vi "(SubVI) Trigger and Record Sine Wave_PI_YCC.vi"(6 "Record time (s)":dbl=0.4, 7 "Amplitude (nm)":dbl=1000.0, 8 "freq. (Hz)":dbl=32.0, 9 "Axis  (Enum)":enum16{"x", "y", "z"}(ring)) -> (0 "Start Position (um)":dbl format="%0.5f", 1 "Read Positions Array (um)":dbl[](array[numeric]), 2 "Target Positions Array (um)":dbl[](array[numeric]), 3 "Time Array (s)":dbl[](array[numeric]), 4 "DAC rate (Hz)":dbl=20000.0)   [LabVIEW 2014]
panel:
  out "Axis Array":i32[](array[numeric])
  out "ADC rate (Hz)":dbl=20000.0
  out "XY Graph":cluster{dbl[], "Data":dbl[]}[](graph)
  out "Xo (Start)":i32
  out "error out":errorcluster
  out "Axis String":string
  out "Axis String Array":string[](array[string])
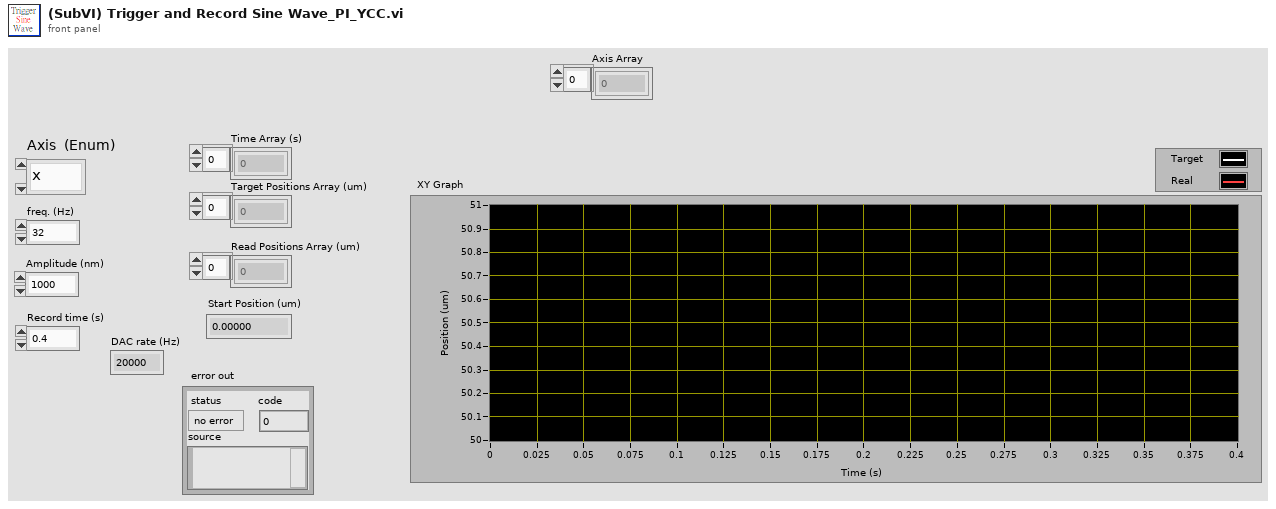
[diagram p1: front panel]
types:
  T1 = cluster{"Time Array (s)":dbl[], "Target Position Array (um)":dbl[]}
  T2 = cluster{"Time Array (s)":dbl[], "Real Position Array (um)":dbl[]}
  T3 = cluster{"Time Array (s)":dbl[], "Real Position Array (um)":dbl[]}[]
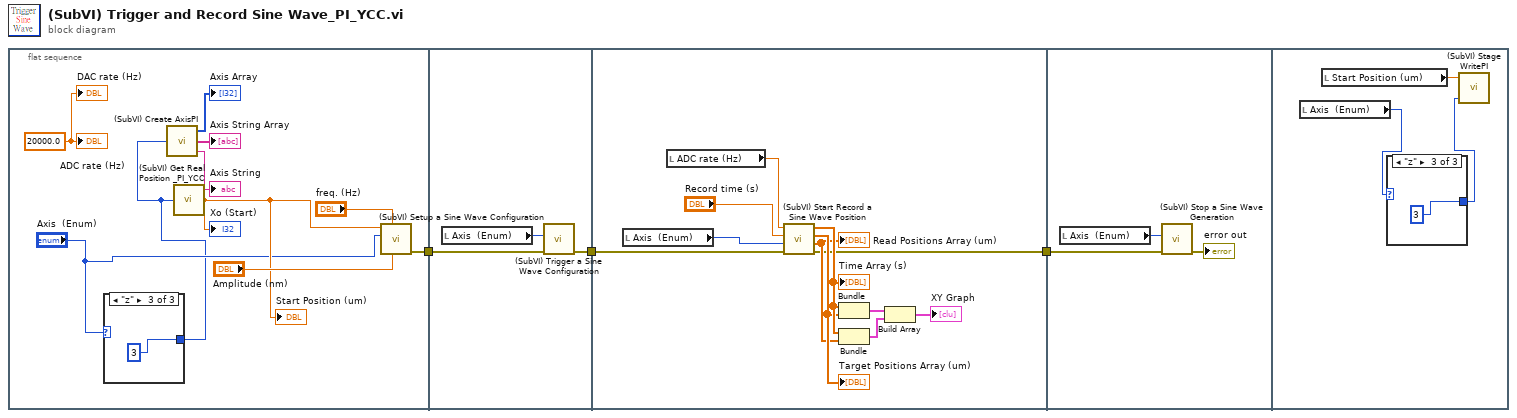
[diagram p0: block diagram]
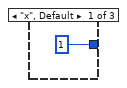
[diagram p2: hidden frame]
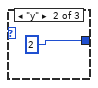
[diagram p3: hidden frame]
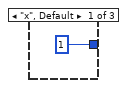
[diagram p4: hidden frame]
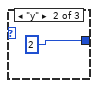
[diagram p5: hidden frame]
diagram:
  n1 = flat-sequence {
    tunnel: [w12] -> w3
    tunnel: w3 -> [w19]
    tunnel: [w18] -> w1
    tunnel: [w23] -> w2
    tunnel: w1 -> [w30]
    tunnel: w2 -> [w33]
    frame #0 {
      w10 = 20000.0 ("x")
      n2 = case shown="\"z\"" "Axis  (Enum)" {
        tunnel: [1 2 3] -> w4
        frame "x", Default {
        }
        frame "y" {
        }
        frame "z" {
        }
      }
      n3 = call "(SubVI) Create AxisPI.vi"("axis"=w4) -> ("Axis String"=→"Axis String":string, "Axis String Array"=→"Axis String Array":string[], "Axis Array"=→"Axis Array":i32[])  [unwired: 2 in]
      n4 = call "(SubVI) Get Real Position _PI_YCC.vi"("Axis"=w4) -> ("Real Current Commanded position (um)"=w9:dbl)  [unwired: 4 in]
      "Xo (Start)" <- w9
      "Start Position (um)" <- w9
      n5 = call "(SubVI) Setup a Sine Wave Configuration.vi"("Amplitude (nm)"="Amplitude (nm)", "freq. (Hz)"="freq. (Hz)", "Axis Enum"="Axis  (Enum)", "Current Commanded position (um)"=w9) -> ("error out"=w12:errorcluster)  [unwired: 7 in]
      "DAC rate (Hz)" <- w10
      "ADC rate (Hz)" <- w10
    }
    frame #1 {
      n6 = local read "Axis  (Enum)"() -> (w17:enum16{"x", "y", "z"})
      n7 = call "(SubVI) Trigger a Sine Wave Configuration.vi"("error in (no error)"=w19, "Axis  (Enum)"=w17) -> ("error out"=w18:errorcluster)  [unwired: 5 in]
    }
    frame #2 {
      n8 = local read "Axis  (Enum)"() -> (w20:enum16{"x", "y", "z"})
      n9 = local read "ADC rate (Hz)"() -> (w21:dbl)
      n10 = call "(SubVI) Start Record a Sine Wave Position.vi"("error in (no error)"=w30, "Axis (Enum)"=w20, "Record time (s)"="Record time (s)", "ADC rate (Hz)"=w21) -> ("error out"=w23:errorcluster, "Real Position Array (um)"=w27:dbl[], "Target Position Array (um)"=w28:dbl[], "Time Array (s)"=w29:dbl[])  [unwired: 4 in]
      "Read Positions Array (um)" <- w27
      "Target Positions Array (um)" <- w28
      "Time Array (s)" <- w29
      n11 = Bundle("Time Array (s)"=w29, "Target Position Array (um)"=w28) -> (w26:T1)  [unwired: 1 in]
      n12 = Bundle("Time Array (s)"=w29, "Real Position Array (um)"=w27) -> (w25:T2)  [unwired: 1 in]
      n13 = Build Array(w26, w25) -> (→"XY Graph":T3)
    }
    frame #3 {
      n14 = local read "Axis  (Enum)"() -> (w31:enum16{"x", "y", "z"})
      n15 = call "(SubVI) Stop a Sine Wave Generation.vi"("error in (no error)"=w33, "Axis  (Enum)"=w31) -> ("error out"=→"error out":errorcluster)  [unwired: 5 in]
    }
    frame #4 {
      n16 = local read "Axis  (Enum)"() -> (w35:enum16{"x", "y", "z"})
      n17 = local read "Start Position (um)"() -> (w36:dbl)
      n18 = case shown="\"z\"" w35 {
        tunnel: [1 2 3] -> w34
        frame "x", Default {
        }
        frame "y" {
        }
        frame "z" {
        }
      }
      n19 = call "(SubVI) Stage WritePI.vi"("axis"=w34, "position"=w36) -> ()  [unwired: 4 in]
    }
  }
